vi "Configure Serial Bus (Flexray - Basic).vi"(0 "VISA resource name":refnum<visa-resource-name>, 1 "Bus Channel (0: A)":i32(ring) items=["A", "B"], 5 "Serial Bus Name (1: Serial Bus 1)":i32(ring)=1 items=["Serial Bus 1"=1, "Serial Bus 2"=2], 9 "Baud Rate (2: 10 Mb/s)":i32(ring)=2 items=["2.5 Mb/s", "5 Mb/s", "10 Mb/s"], 11 "error in (no error)":errorcluster, 12 "Source (0: Channel 1)":i32(ring) items=["Channel 1", "Channel 2", "Channel 3", "Channel 4"]) -> (4 "VISA resource name out":refnum<visa-resource-name>, 15 "error out":errorcluster)   [LabVIEW 2015, in "Agilent 2000 3000 X-Series.lvlib"]
doc: "Configures the basic settings of FlexRay bus.\n\nNote:\nThis VI is not supported by EDUX1052A/G, DSOX1202A/G, DSOX1204A/G models"
uses:
  Agilent 2000 3000 X-Series.lvlib
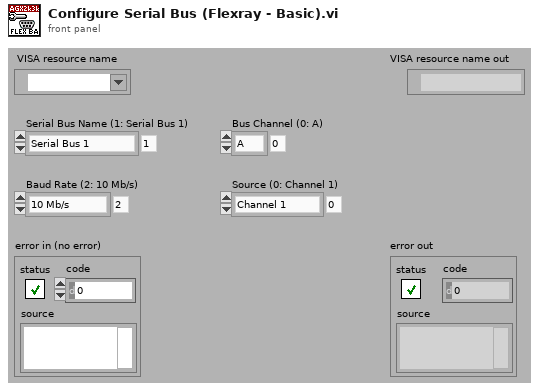
[diagram p1: front panel]
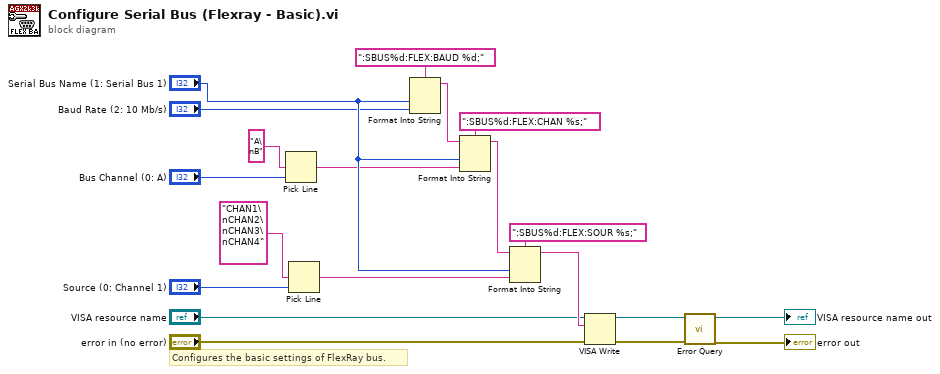
[diagram p0: block diagram]
diagram:
  # "Configures the basic settings of FlexRay bus."
  n1 = Pick Line(multi-line string="A\nB", line index="Bus Channel (0: A)") -> (output string=w13:string)  [unwired: 1 out]
  n2 = Pick Line(multi-line string="CHAN1\nCHAN2\nCHAN3\nCHAN4", line index="Source (0: Channel 1)") -> (output string=w8:string)  [unwired: 1 out]
  n3 = Format Into String(format string=":SBUS%d:FLEX:BAUD %d;", "Serial Bus Name (1: Serial Bus 1)", "Baud Rate (2: 10 Mb/s)") -> (resulting string=w15:string)  [unwired: 2 in, 1 out]
  n4 = Format Into String(format string=":SBUS%d:FLEX:CHAN %s;", initial string=w15, "Serial Bus Name (1: Serial Bus 1)", w13) -> (resulting string=w10:string)  [unwired: 1 in, 1 out]
  n5 = Format Into String(format string=":SBUS%d:FLEX:SOUR %s;", initial string=w10, "Serial Bus Name (1: Serial Bus 1)", w8) -> (resulting string=w7:string)  [unwired: 1 in, 1 out]
  n6 = VISA Write(VISA resource name="VISA resource name", write buffer=w7, error in (no error)="error in (no error)") -> (VISA resource name out=w4:refnum<visa-resource-name>, error out=w3:errorcluster)  [unwired: 1 out]
  n7 = call "Error Query.vi"("error in (no error)"=w3, "VISA resource name"=w4) -> ("error out"=→"error out":errorcluster, "VISA resource name out"=→"VISA resource name out":refnum<visa-resource-name>)  [unwired: 8 out]
